vi "Aggregate Test Case Results.vi"(10 "Test Case Result":T1, 11 "Test Suite Result In":T6) -> (3 "Test Suite Result Out":T6)   [LabVIEW 2020, in "Test Suite Result.lvlib"]
uses:
  Test Suite Result.lvlib
  Test Suite Result.ctl
  Assertion Result/Public/TypeDefs/Status.ctl
  Case Result/Test Case Result.ctl
  Method Result/Method Result.ctl
  Rewrite Project/Result/Status.ctl
  Assertion Result/Assertion Result.ctl
  Assertion Result/Public/TypeDefs/Assertion Type.ctl
  Case Result/Test Case Result.lvlib
  Assertion Result/Assertion Result.lvlib
  Method Result/Method Result.lvlib
  Rewrite Project/Result/Result.lvlib
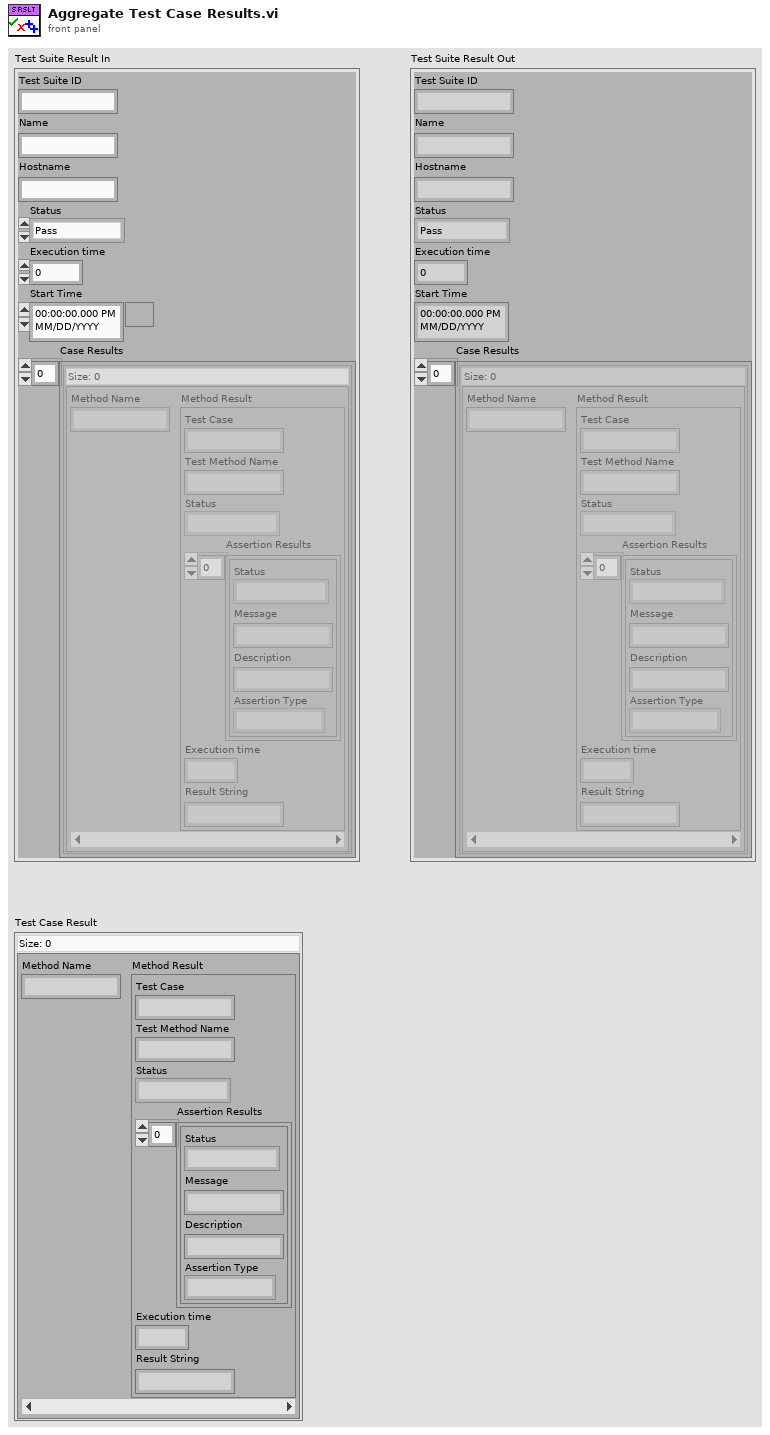
[diagram p1: front panel]
types:
  T1 = typedef "Test Case Result.lvlib/Test Case Result.ctl" = map{string, T2}
  T2 = typedef "Method Result.lvlib/Method Result.ctl" = cluster{"Test Case":string, "Test Method Name":string, "Status":T3, "Assertion Results":T4[], "Execution time":dbl, "Result String":string}
  T3 = typedef "Result.lvlib/Status.ctl" = enum16{"Pass", "Fail", "Error", "Skipped", "Setup Error", "Broken", "Teardown Error"}
  T4 = typedef "Assertion Result.lvlib/Assertion Result.ctl" = cluster{"Status":T3, "Message":string, "Description":string, "Assertion Type":T5}
  T5 = typedef "Result.lvlib/Assertion Type.ctl" = enum16{"None", "Pass", "Fail", "Skip", "Pass if Equal", "Fail if Equal", "Pass if Error", "Fail if Error", "Pass if", "Fail if"}
  T6 = typedef "Test Suite Result.lvlib/Test Suite Result.ctl" = cluster{"Test Suite ID":string, "Name":string, "Hostname":string, "Status":T7, "Execution time":dbl, "Start Time":timestamp, "Case Results":T1[]}
  T7 = typedef "Assertion Result.lvlib/Status.ctl" = enum16{"Pass", "Fail", "Error", "Skipped", "Setup Error", "Broken", "Teardown Error"}
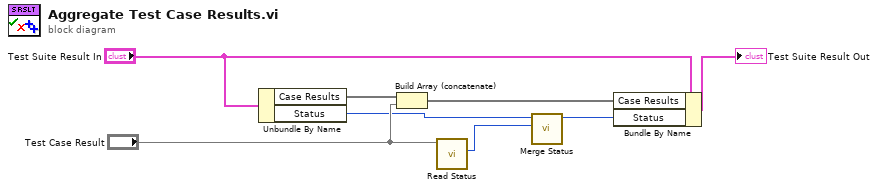
[diagram p0: block diagram]
diagram:
  n1 = Unbundle By Name("Test Suite Result In") -> ("Case Results"=w5:T1[], "Status"=w2:T7)
  n2 = Build Array (concatenate)(w5, "Test Case Result") -> (w4:T1[])
  n3 = call "Read Status.vi"("Test Case Result In"="Test Case Result") -> ("Status"=w1:T7)  [unwired: 8 in, 2 out]
  n4 = call "Merge Status.vi"("New"=w1, "Current"=w2) -> ("Merged"=w3:T7)  [unwired: 8 in, 1 out]
  n5 = Bundle By Name(cluster="Test Suite Result In", "Case Results"=w4, "Status"=w3) -> (→"Test Suite Result Out":T6)
